vi "get_wavelength.vi"(8 "error in (no error)":errorcluster, 11 "LightSourceMH110124MaiTai in":refnum<class "LightSourceMH110124MaiTai.lvclass">) -> (0 "error out":errorcluster, 2 "wavelength":dbl[unit], 3 "LightSourceMH110124MaiTai out":refnum<class "LightSourceMH110124MaiTai.lvclass">)   [LabVIEW 2010, in "LightSourceMH110124MaiTai.lvclass"]
uses:
  LightSourceMH110124MaiTai.lvclass
  LightSourceMH110124MaiTai.lvclass/LightSourceMH110124MaiTai.ctl
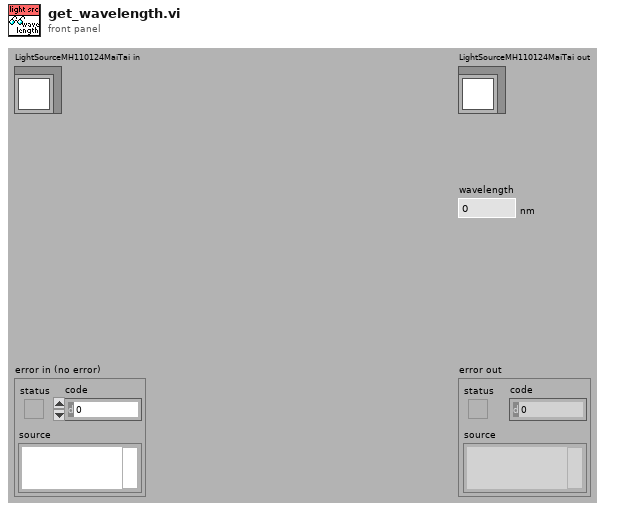
[diagram p1: front panel]
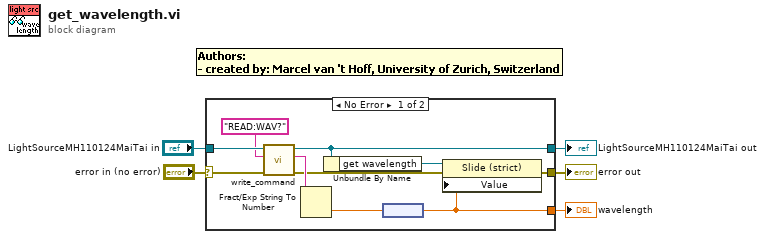
[diagram p0: block diagram]
diagram:
  n1 = case shown="No Error" "error in (no error)" {
    selector: "error in (no error)" -> [w14 w17]
    tunnel: "LightSourceMH110124MaiTai in" -> [w15 w16]
    tunnel: [w11 w16] -> w4
    tunnel: [w8 w17] -> w2
    tunnel: [w6 _] -> w1
    frame No Error {
      n2 = call-dynamic "write_command.vi"("error in (no error)"=w14, "string to write"="READ:WAV?", "LightSourceMH110124MaiTai in"=w15) -> ("error out"=w9:errorcluster, "read string"=w13:string, "LightSourceMH110124MaiTai out"=w11:refnum<class "LightSourceMH110124MaiTai.lvclass">)  [unwired: 6 in]
      n3 = Fract/Exp String To Number(string=w13) -> (number=w7:dbl)  [unwired: 3 in, 1 out]
      n4 = Unbundle By Name(w11) -> ("get wavelength"=w10:refnum<vi>)
      n5 = node(w7) -> (w6:dbl[unit])
      n6 = property class="Slide (strict)"(reference=w10, error in=w9, "Value"=w6) -> (error out=w8:errorcluster)  [unwired: 1 out]
    }
    frame Error {
    }
  }
  "error out" <- w2
  "LightSourceMH110124MaiTai out" <- w4
  "wavelength" <- w1
